vi "Generic Client FGV.vi"(8 "error in":errorcluster, 9 "unique id in":u64, 10 "action":T3, 11 "vi references in":T1) -> (0 "error out":errorcluster, 1 "unique id out":u64, 2 "grpc client id":T2)   [LabVIEW 2020, in "MeasurementLink gRPC Utilities.lvlib"]
uses:
  MeasurementLink gRPC Utilities.lvlib
  <vilib>/gRPC/LabVIEW gRPC Library/Shared/grpcId.ctl
  <vilib>/gRPC/LabVIEW gRPC Library/grpc-lvsupport-release.lvlib
  Action.ctl
  VI References.ctl
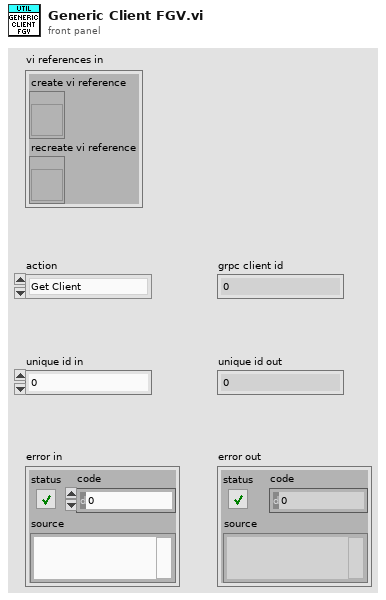
[diagram p1: front panel]
types:
  T1 = typedef "MeasurementLink gRPC Utilities.lvlib/VI References.ctl" = cluster{"create vi reference":refnum<vi>, "recreate vi reference":refnum<vi>}
  T2 = typedef "grpc-lvsupport-release.lvlib/grpcId.ctl" = u64
  T3 = typedef "MeasurementLink gRPC Utilities.lvlib/Action.ctl" = enum16{"Get Client", "Recreate Client"}
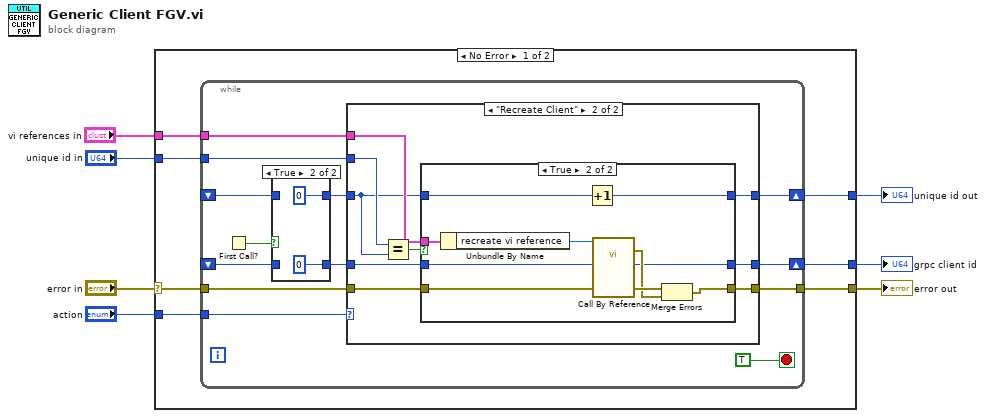
[diagram p0: block diagram]
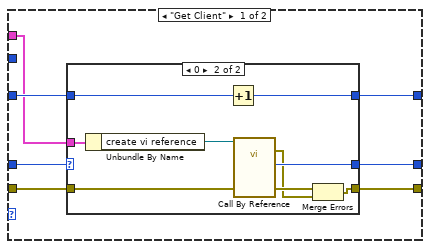
[diagram p3: hidden frame]
diagram:
  n1 = case shown="No Error" "error in" {
    selector: "error in" -> [w13 w73]
    tunnel: [w12 w73] -> w7
    tunnel: "action" -> [w14 _]
    tunnel: [w11 _] -> w6
    tunnel: [w10 _] -> w5
    tunnel: "unique id in" -> [w9 _]
    tunnel: "vi references in" -> [w8 _]
    frame No Error {
      n2 = while {
        tunnel: w14 -> [w26]
        tunnel: w13 -> [w25]
        tunnel: [w24] -> w12
        shift-right: [w23] -> w11
        shift-left: _ -> [w21]
        shift-right: [w17] -> w10
        shift-left: _ -> [w19]
        tunnel: w9 -> [w16]
        tunnel: w8 -> [w15]
        stop <- TRUE stop-if-true
        n3 = First Call?() -> (First Call?: T/F=w22:bool)
        n4 = case shown="True" w22 {
          tunnel: w21 -> [w29 _]
          tunnel: [w29 T2 0 ("gRPC ID out")] -> w20
          tunnel: w19 -> [w28 _]
          tunnel: [w28 u64 0] -> w18
          frame False {
          }
          frame True {
          }
        }
        n5 = case shown="\"Recreate Client\"" w26 {
          tunnel: w25 -> [w35 w57]
          tunnel: [w38 w58] -> w24
          tunnel: [w37 w54] -> w23
          tunnel: w20 -> [w36 w59]
          tunnel: w18 -> [w34 w52]
          tunnel: [w33 w51] -> w17
          tunnel: w16 -> [_ w56]
          tunnel: w15 -> [w32 w53]
          frame "Get Client" {
            n6 = case shown="0" w36 {
              selector: w36 -> [w41 _]
              tunnel: w35 -> [w40 w47]
              tunnel: [w40 w42] -> w38
              tunnel: [w41 w45] -> w37
              tunnel: w34 -> [w39 w50]
              tunnel: [w39 w49] -> w33
              tunnel: w32 -> [_ w46]
              frame Default {
              }
              frame 0 {
                n7 = Unbundle By Name(w46) -> ("create vi reference"=w48:refnum<vi>)
                n8 = Increment(x=w50) -> (x+1=w49:u64)
                n9 = call-by-ref "?"(reference=w48, "error in"=w47) -> (error out=w43:errorcluster, 0:"error out"=w44:errorcluster, "grpc client id"=w45:T2)  [unwired: 10 in, 1 out]
                n10 = Merge Errors(w44, w43) -> (w42:errorcluster)
              }
            }
          }
          frame "Recreate Client" {
            n11 = Equal?(x=w56, y=w52) -> (x = y?=w55:bool)
            n12 = case shown="True" w55 {
              tunnel: w59 -> [w61 w70]
              tunnel: [w62 w66] -> w58
              tunnel: w57 -> [w62 w69]
              tunnel: [w61 w65] -> w54
              tunnel: w53 -> [_ w72]
              tunnel: w52 -> [w60 w64]
              tunnel: [w60 w63] -> w51
              frame False {
              }
              frame True {
                n13 = Unbundle By Name(w72) -> ("recreate vi reference"=w71:refnum<vi>)
                n14 = Increment(x=w64) -> (x+1=w63:u64)
                n15 = call-by-ref "?"(reference=w71, "error in"=w69, "grpc client id in"=w70) -> (error out=w67:errorcluster, 0:"error out"=w68:errorcluster, "grpc client id out"=w65:T2)  [unwired: 9 in, 1 out]
                n16 = Merge Errors(w68, w67) -> (w66:errorcluster)
              }
            }
          }
        }
      }
    }
    frame Error {
    }
  }
  "error out" <- w7
  "grpc client id" <- w6
  "unique id out" <- w5
